vi "Diagnostics.Main.UUDT.Engine.vi"(8 "error in (no error)":errorcluster, 11 "State Variables":T1={"Comm"=refnum, "Parameters"={"Name"="", "CAN"={"Interface"="", "Baud Rate"=0, "Diagnostic Protocol"=enum."GMLAN", "Transport Protocol"=enum."ISO TP - Normal Mode", "Transmit ID"=0, "Receive ID"=2, "Transmit Extension"=1, "Receive Extension"=255, "Receive UUDT ID"=0, "Enable Stream"=TRUE, "VW TP Channel ID"=1, "Fill Frame"=FALSE, "Fill Byte"=0, "Termination"=FALSE, "LIN Cluster"="", "NAD"=8, "IO Mode"=0, "Max DLC"=0, "FD Baud Rate"=2, "Timeout"=1}, "986x"={"Enable"=FALSE, "RIO Device"="", "Bitfile"=path ""}, "Reads"=[], "Frames Lookup"=variant(enum16{"GMLAN", "KWP-2000", "UDS"} enum."GMLAN"), "Writes"=[], "DPIDs"=[], "DPID Lookup"=variant(u32 0), "DTC"={"Descriptor"={"DTC Byte Length"=1, "Status Byte Length"=1, "Add Data Byte Length"=1, "Byte Order"=enum."Motorola"}, "Value.Code"=[], "Value.String"=[], "Value.J2012String"=[], "Status.Code"=[], "Status.String"=[]}, "Created DTCs"=0, "Polls"=[], "Service Channels Status Lookup"=variant, "Trigger Lookup"=variant, "Security"={"Type"=enum."None", "Source DLL Path"=path "", "Target DLL Path"=path "", "Security Level"=0}}, "ADCS Connection"={"Diag CAN Handle"=0, "Transport Protocol"=enum."ISO TP - Normal Mode", "Receive Address Extension"=0, "Transmit Address Extension"=0, "Receive CAN Id"=0, "Transmit CAN Id"=0, "Log Frames ?"=FALSE, "My TP Address"=0, "Other TP Address"=0, "T1"=0, "T2"=0, "T3"=0, "T4"=0, "Tx SN"=0, "Block Size"=0, "Rx SN"=0, "VW TP Initialized?"=FALSE, "Tx block no"=0, "baud rate"=0, "Interface"="", "Channel Diag CAN Handle"=0, "UDP Connection ID"=refnum, "TCP Connection ID"=refnum, "Target IP Addr"=0, "Source Address"=0, "Target Address"=0, "Send Header NACK?"=FALSE, "DLL Handle"=0, "NAD"=0, "Time Stamp read first"=0.0, "Time Stamp read last"=0.0, "Time Stamp write first"=0.0, "Time Stamp write last"=0.0, "Time Stamp write"=0.0, "Time Stamp read"=0.0, " I/O Mode"=0, "FD Baudrate"=0, "TX_DL"=8, "RX_DL"=8, "DoIP Protocol Version"=1, " Selected I/O Mode"=0, "TesterPresent Counter"=0, "TesterPresent Limit"=0, "TesterPresent Tick[ms]"=10, "TesterPresent RequireResponse?"=FALSE, "TesterPresent Stored Ref?"=FALSE, "TesterPresent Message"=[], "TesterPresent Task Handle"=0, "TesterPresent Semaphore"=refnum, "Response Plausibility Check"=1, "Default Version?"=TRUE, "Diagostic Globals"={"Timeout FC (Bs)"=250, "Timeout CF (Cr)"=250, "Timeout Diag Command"=1000, "Receive Block Size (BS)"=0, "Wait Time CF (STmin)"=5, "Max Waits (N_WFTmax)"=10, "Waits to Send (N_WAIT)"=0, "Time between Waits (TW)"=25, "Fill CAN Frames?"=TRUE, "Fill Byte"=255, "Invalid Response as Error?"=FALSE, "Max RspPending Count"=5, "VWTP Command Timeout"=50, "Transport Protocol"=enum."Diagnostics on IP", "Diag CAN Handle"=0, "DLL Handle"=0, "Timeout RspPending"=1000}, "Session-based Properties?"=FALSE}, "XNET References"={"Database"="", "GMLAN DPID Session"="", "Cluster"=""}, "XNETEngine (GMLAN)"=refnum, "Process"=refnum, "Reads"=refnum, "Writes"=refnum, "Cmds"=refnum, "DTCs"=refnum, "DTC Count"=refnum, "Status"=refnum, "Triggers"=refnum, "CANConnected"=refnum, "LocalStop"=refnum, "LocalCommStatus"=refnum, "Service Channels Status"=refnum, "Settings"=refnum} {"ADCS Connection"."Diagostic Globals"."Fill Byte" format="%x"; "ADCS Connection"."TesterPresent Message" format="%.0x"; "ADCS Connection"."Selected I/O Mode" items=["CAN", "CAN FD", "CAN FD+BRS", "ECU Determined"]; "ADCS Connection"."DoIP Protocol Version" items=["2010"=1, "2012"=2]; "ADCS Connection"."RX_DL" items=["8"=8, "12"=12, "16"=16, "20"=20, "24"=24, "32"=32, "48"=48, "64"=64]; "ADCS Connection"."TX_DL" items=["8"=8, "12"=12, "16"=16, "20"=20, "24"=24, "32"=32, "48"=48, "64"=64]; "ADCS Connection"."I/O Mode" items=["CAN", "CAN FD", "CAN FD+BRS", "Not yet determined"]; "Parameters"."Writes"."Signals"."Byte Order" items=["Little Endian", "Big Endian"]; "Parameters"."Writes"."Signals"."Data Type" items=["Signed", "Unsigned", "IEEE Float"]; "Parameters"."CAN"."IO Mode" items=["CAN 2.0", "CAN FD", "CAN FD+BRS"]; "Parameters"."CAN"."Fill Byte" format="%.0x"; "Parameters"."CAN"."VW TP Channel ID" format="%.0x"; "Parameters"."CAN"."Receive UUDT ID" format="%.0x"; "Parameters"."CAN"."Receive Extension" format="%.0x"; "Parameters"."CAN"."Transmit Extension" format="%.0x"; "Parameters"."CAN"."Receive ID" format="%.0x"; "Parameters"."CAN"."Transmit ID" format="%.0x"; "Parameters"."Reads"."Signals"."Byte Order" items=["Little Endian", "Big Endian"]; "Parameters"."Reads"."Signals"."Data Type" items=["Signed", "Unsigned", "IEEE Float"]}) -> (0 "error out":errorcluster)   [LabVIEW 2019, in "Diagnostics Addon Engine.lvlib"]
uses:
  Diagnostics Addon Engine.lvlib
  Types/Diagnostics.State.ctl
  <vilib>/NI/NIVS Inline Async API/_VS Inline Async API/Process/Process.lvclass
  <vilib>/NI/NI VeriStand Addon Network Comm/Engine/VeriStand Comm.lvclass
  Addon Shared/Types/SysDef.Compile.ctl
  Addon Shared/Types/CAN.ctl
  Addon Shared/Types/CAN.Interface.ctl
  Addon Shared/Types/Protocol.ctl
  Addon Shared/Types/Transport.ctl
  Addon Shared/Types/986x.ctl
  Addon Shared/Types/Frame.Compile.ctl
  Addon Shared/Types/Type.ctl
  Addon Shared/Types/Signal.ctl
  Addon Shared/Types/DPID.ctl
  Addon Shared/Types/DPID.Rate.ctl
  Addon Shared/Types/DTC.Settings.ctl
  Addon Shared/Types/DTC.Descriptor.ctl
  Addon Shared/Types/Poll.Compiled.ctl
  Addon Shared/Types/Security.ctl
  Addon Shared/Types/Security.Type.ctl
  <vilib>/Automotive Diagnostic Command Set/Diagnostic Transport.llb/Diag Reference.ctl
  <vilib>/Automotive Diagnostic Command Set/Diagnostic Transport.llb/Transport Protocol Selector.ctl
  <vilib>/Automotive Diagnostic Command Set/Diagnostic Transport.llb/DoIP Protocol Version.ctl
  <vilib>/Automotive Diagnostic Command Set/Diagnostic Transport.llb/Diag Globals.ctl
  Types/XNET.Refs.ctl
  <vilib>/NI/AMC/Message Queue.ctl
  <vilib>/NI/AMC/Message.ctl
  <vilib>/NI/Tools/Keyed Array/KeyedArray.ctl
  <vilib>/NI/NIVS Inline Async API/_Data Access Engine/Data Access Engine/Types/Write.DVR.ctl
  <vilib>/NI/NIVS Inline Async API/_Data Access Engine/Access Type Classes/Write/Write.lvclass
  <vilib>/NI/NIVS Inline Async API/_Data Access Engine/Data Access Engine/Types/Read.DVR.ctl
  <vilib>/NI/NIVS Inline Async API/_Data Access Engine/Access Type Classes/Read/Read.lvclass
  <vilib>/NI/NIVS Inline Async API/_Data Access Engine/Data Access Engine/Types/ReadWrite.DVR.ctl
  <vilib>/NI/NIVS Inline Async API/_Data Access Engine/Access Type Classes/ReadWrite/ReadWrite.lvclass
  Addon Shared/Types/DTC.Info.ctl
  Types/DTC.ChangeCount.Info.ctl
  <vilib>/xnet/xnet.llb/XNET Frame CAN.ctl
  <vilib>/xnet/xnet.llb/XNET Frame Type CAN.ctl
  <vilib>/NI/NIVS Inline Async API/_Data Access Engine/Access Type Classes/Write/Write.lvclass/Write.ctl
  Addon Shared/Types/Frame.Data.ctl
  Addon Shared/Types/DPID.Lookup.Info.ctl
  Addon Shared/Types/DPID.Lookup.Info.PID.ctl
  <vilib>/NI/NI VeriStand Addon Network Comm/Engine/VeriStand Comm.lvclass/VeriStand Comm.ctl
  <vilib>/NI/NIVS Inline Async API/_VS Inline Async API/Process/Process.lvclass/Process.ctl
  <vilib>/NI/NIVS Inline Async API/_Data Access Engine/Data Access Engine/Methods/Write.Data.vi
  <vilib>/NI/NIVS Inline Async API/_Data Access Engine/Data Access Engine/Methods/Write.Data.Commit.vi
  <vilib>/NI/NIVS Inline Async API/_Data Access Engine/Access Type Classes/Write/Write.ProcessData.vi
  <vilib>/NI/NIVS Inline Async API/_Data Access Engine/Data Access Engine/Methods/Write.Data.Buffer.vi
  Addon Shared/SubVIs/LookupID.Create.vi
  <vilib>/NI/NIVS Inline Async API/_Data Access Engine/Access Type Classes/Write/Write.Commit.vi
  Support Libraries/GMLAN/Utilities/Convert Raw Data to DTCs.vi
  <vilib>/NI/AMC/Send Local Message.vi
  <vilib>/NI/AMC/Read Termination Message.vi
  <vilib>/NI/NIVS Inline Async API/_VS Inline Async API/Error Handling Process/SubVIs/Error.ConvertArray.vi
  <vilib>/NI/NIVS Inline Async API/_Data Access Engine/Access Type Classes/Write/Write.Buffer.vi
  <vilib>/NI/AMC/Create Single Message.vi
  <vilib>/NI/AMC/Update Message Routing Info.vi
  <vilib>/NI/AMC/Globals.vi
  Addon Shared/SubVIs/Constants.vi
  <vilib>/Utility/SystemLogging/Write to System Log.vi
  <vilib>/xnet/xnet.llb/XNET Convert.vi
  <vilib>/xnet/xnet.llb/XNET Convert (Frame CAN to Signal).vi
  <vilib>/xnet/xnet.llb/XNET Read (Frame CAN).vi
  <vilib>/Automotive Diagnostic Command Set/Diagnostic Protocols.llb/Convert to Phys.vi
  <vilib>/NI/AMC/Send Message.vi
  Addon Shared/Diagnostics Addon Shared.lvlib
  <vilib>/NI/AMC/AMC.lvlib
  Support Libraries/GMLAN/GMLAN.lvlib
  <vilib>/NI/NIVS Inline Async API/_Data Access Engine/Data Access Engine/Data Access Engine.lvclass
  <vilib>/NI/Tools/Keyed Array/Tools_KeyedArray.lvlib
  <vilib>/addons/Automotive Diagnostic Command Set/NI_Automotive Diagnostic Command Set.lvlib
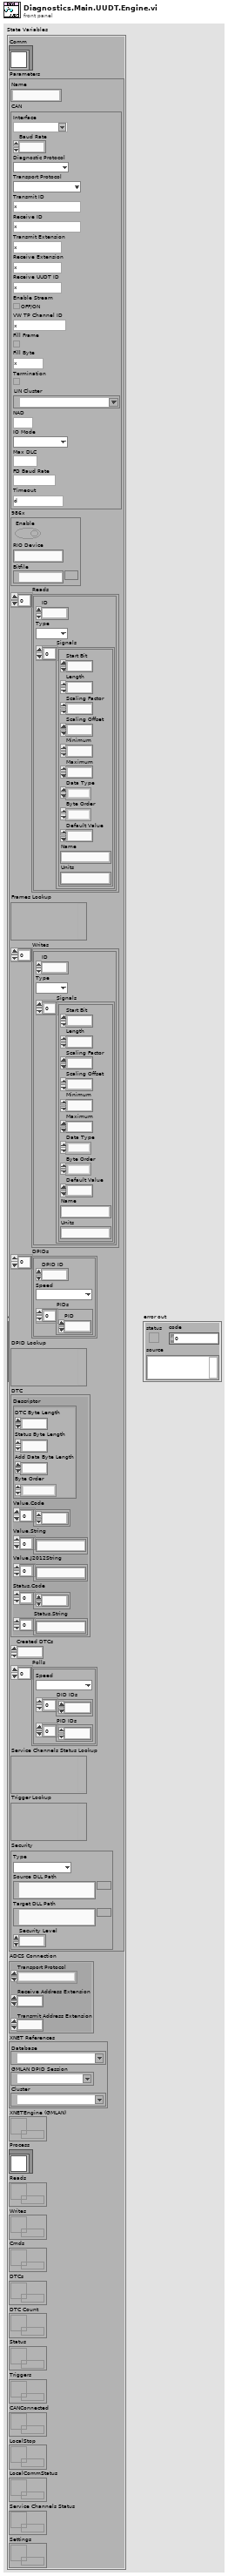
[diagram p1: front panel]
types:
  T1 = typedef "Diagnostics Addon Engine.lvlib/Diagnostics.State.ctl" = cluster{"Comm":refnum<class "VeriStand Comm.lvclass">, "Parameters":T2, "ADCS Connection":T18, "XNET References":T23, "XNETEngine (GMLAN)":T24, "Process":refnum<class "Process.lvclass">, "Reads":T25, "Writes":T26, "Cmds":T27, "DTCs":T25, "DTC Count":T25, "Status":T25, "Triggers":T27, "CANConnected":T25, "LocalStop":refnum<data-value>, "LocalCommStatus":refnum<data-value>, "Service Channels Status":T25, "Settings":T26}
  T2 = typedef "Diagnostics Addon Shared.lvlib/SysDef.Compile.ctl" = cluster{"Name":string, "CAN":T3, "986x":T7, "Reads":T8[], "Frames Lookup":variant, "Writes":T8[], "DPIDs":T11[], "DPID Lookup":variant, "DTC":T13, "Created DTCs":u32, "Polls":T15[], "Service Channels Status Lookup":variant, "Trigger Lookup":variant, "Security":T16}
  T3 = typedef "Diagnostics Addon Shared.lvlib/CAN.ctl" = cluster{"Interface":T4, "Baud Rate":u64, "Diagnostic Protocol":T5, "Transport Protocol":T6, "Transmit ID":u32, "Receive ID":u32, "Transmit Extension":u8, "Receive Extension":u8, "Receive UUDT ID":u32, "Enable Stream":bool, "VW TP Channel ID":u32, "Fill Frame":bool, "Fill Byte":u8, "Termination":bool, "LIN Cluster":refnum<k21>, "NAD":u8, "IO Mode":u32, "Max DLC":u16, "FD Baud Rate":u64, "Timeout":u32}
  T4 = typedef "Diagnostics Addon Shared.lvlib/CAN.Interface.ctl" = string
  T5 = typedef "Diagnostics Addon Shared.lvlib/Protocol.ctl" = enum16{"GMLAN", "KWP-2000", "UDS", "User-Defined"}
  T6 = typedef "Diagnostics Addon Shared.lvlib/Transport.ctl" = enum16{"ISO TP - Normal Mode", "ISO TP - Mixed Mode", "VW TP 2.0", "Diagnostics on IP", "ISO TP LIN"}
  T7 = typedef "Diagnostics Addon Shared.lvlib/986x.ctl" = cluster{"Enable":bool, "RIO Device":string, "Bitfile":path}
  T8 = typedef "Diagnostics Addon Shared.lvlib/Frame.Compile.ctl" = cluster{"ID":u32, "Type":T9, "Signals":T10[]}
  T9 = typedef "Diagnostics Addon Shared.lvlib/Type.ctl" = enum16{"DID", "CDID", "PID", "CPID", "Read Memory", "Write Memory", "IO Control", "Routine Start", "Routine Request", "Routine Stop", "User Defined", "DTC Control", "Clear DTCs", "Read DTCs", "Start DTCs", "DTC Change Count", "Tester Present", "Unlock ECU", "Reset ECU", "Diag Session Control", "Communication Control", "DPID Control", "Poll Control", "Diag CAN Control"}
  T10 = typedef "Diagnostics Addon Shared.lvlib/Signal.ctl" = cluster{"Start Bit":u32, "Length":u32, "Scaling Factor":dbl, "Scaling Offset":dbl, "Minimum":dbl, "Maximum":dbl, "Data Type":u32, "Byte Order":u32, "Default Value":dbl, "Name":string, "Units":string}
  T11 = typedef "Diagnostics Addon Shared.lvlib/DPID.ctl" = cluster{"DPID ID":u8, "Speed":T12, "PIDs":u16[]}
  T12 = typedef "Diagnostics Addon Shared.lvlib/DPID.Rate.ctl" = enum16{"Slow", "Medium", "Fast"}
  T13 = typedef "Diagnostics Addon Shared.lvlib/DTC.Settings.ctl" = cluster{"Descriptor":T14, "Value.Code":dbl[], "Value.String":string[], "Value.J2012String":string[], "Status.Code":dbl[], "Status.String":string[]}
  T14 = typedef "Diagnostics Addon Shared.lvlib/DTC.Descriptor.ctl" = cluster{"DTC Byte Length":i32, "Status Byte Length":i32, "Add Data Byte Length":i32, "Byte Order":enum16{"Motorola", "Intel"}}
  T15 = typedef "Diagnostics Addon Shared.lvlib/Poll.Compiled.ctl" = cluster{"Speed":T12, "DID IDs":u32[], "PID IDs":u32[]}
  T16 = typedef "Diagnostics Addon Shared.lvlib/Security.ctl" = cluster{"Type":T17, "Source DLL Path":path, "Target DLL Path":path, "Security Level":u8}
  T17 = typedef "Diagnostics Addon Shared.lvlib/Security.Type.ctl" = enum16{"None", "DLL", "MasterKey"}
  T18 = typedef "NI_Automotive Diagnostic Command Set.lvlib/Diag Reference.ctl" = cluster{"Diag CAN Handle":u32, "Transport Protocol":T19, "Receive Address Extension":u8, "Transmit Address Extension":u8, "Receive CAN Id":u32, "Transmit CAN Id":u32, "Log Frames ?":bool, "My TP Address":u8, "Other TP Address":u8, "T1":u16, "T2":u16, "T3":u16, "T4":u16, "Tx SN":u8, "Block Size":u8, "Rx SN":u8, "VW TP Initialized?":bool, "Tx block no":u8, "baud rate":u64, "Interface":string, "Channel Diag CAN Handle":u32, "UDP Connection ID":refnum<k16>, "TCP Connection ID":refnum<k5>, "Target IP Addr":u32, "Source Address":u16, "Target Address":u16, "Send Header NACK?":bool, "DLL Handle":u32, "NAD":u8, "Time Stamp read first":dbl, "Time Stamp read last":dbl, "Time Stamp write first":dbl, "Time Stamp write last":dbl, "Time Stamp write":dbl, "Time Stamp read":dbl, " I/O Mode":u32, "FD Baudrate":u64, "TX_DL":u16, "RX_DL":u16, "DoIP Protocol Version":T20, " Selected I/O Mode":u32, "TesterPresent Counter":u32, "TesterPresent Limit":u32, "TesterPresent Tick[ms]":i32, "TesterPresent RequireResponse?":bool, "TesterPresent Stored Ref?":bool, "TesterPresent Message":u8[], "TesterPresent Task Handle":i32, "TesterPresent Semaphore":T21, "Response Plausibility Check":u32, "Default Version?":bool, "Diagostic Globals":T22, "Session-based Properties?":bool}
  T19 = typedef "NI_Automotive Diagnostic Command Set.lvlib/Transport Protocol Selector.ctl" = enum16{"ISO TP - Normal Mode", "ISO TP - Mixed Mode", "VW TP 2.0", "Diagnostics on IP", "ISO TP LIN"}
  T20 = typedef "NI_Automotive Diagnostic Command Set.lvlib/DoIP Protocol Version.ctl" = u8
  T21 = typedef "Semaphore RefNum" = refnum<k1>
  T22 = typedef "NI_Automotive Diagnostic Command Set.lvlib/Diag Globals.ctl" = cluster{"Timeout FC (Bs)":u32, "Timeout CF (Cr)":u32, "Timeout Diag Command":u32, "Receive Block Size (BS)":u8, "Wait Time CF (STmin)":u8, "Max Waits (N_WFTmax)":u8, "Waits to Send (N_WAIT)":i32, "Time between Waits (TW)":u32, "Fill CAN Frames?":bool, "Fill Byte":u32, "Invalid Response as Error?":bool, "Max RspPending Count":u32, "VWTP Command Timeout":u32, "Transport Protocol":T19, "Diag CAN Handle":u32, "DLL Handle":u32, "Timeout RspPending":u32}
  T23 = typedef "Diagnostics Addon Engine.lvlib/XNET.Refs.ctl" = cluster{"Database":refnum<k21>, "GMLAN DPID Session":refnum<k21>, "Cluster":refnum<k21>}
  T24 = typedef "AMC.lvlib/Message Queue.ctl" = refnum<queue>
  T25 = typedef "Data Access Engine.lvlib/Data Access Engine.lvclass/Write.DVR.ctl" = refnum<data-value>
  T26 = typedef "Data Access Engine.lvlib/Data Access Engine.lvclass/Read.DVR.ctl" = refnum<data-value>
  T27 = typedef "Data Access Engine.lvlib/Data Access Engine.lvclass/ReadWrite.DVR.ctl" = refnum<data-value>
  T28 = typedef "Diagnostics Addon Shared.lvlib/DTC.Info.ctl" = cluster{"Timestamp":dbl, "DTC":dbl, "Status":dbl, "Add Data":dbl}
  T29 = typedef "Diagnostics Addon Engine.lvlib/DTC.ChangeCount.Info.ctl" = cluster{"DTCCountChange?":bool, "Timestamp":timestamp}
  T30 = typedef "XNET Frame CAN.ctl" = cluster{"timestamp":timestamp, "payload":u8[], "identifier":u32, "type":T31, "extended?":bool, "echo?":bool}
  T31 = typedef "XNET Frame Type CAN.ctl" = u8
  T32 = cluster{"Change DTC Count Cluster":T29, "Previous DTCs":T28[], "Prev DTC Frames":T30[]}
  T33 = typedef "Diagnostics Addon Shared.lvlib/Frame.Data.ctl" = cluster{"ID":u32, "Raw Frame":u8[], "error out":errorcluster}
  T34 = typedef "Diagnostics Addon Shared.lvlib/DPID.Lookup.Info.ctl" = cluster{"PID Info":T35}
  T35 = typedef "Diagnostics Addon Shared.lvlib/DPID.Lookup.Info.PID.ctl" = cluster{"PID":u16, "Frame Length":u8}
  T36 = typedef "Diagnostic Trouble Code.ctl" = cluster{"DTC":u32, "Status":u32, "Add Data":u32}
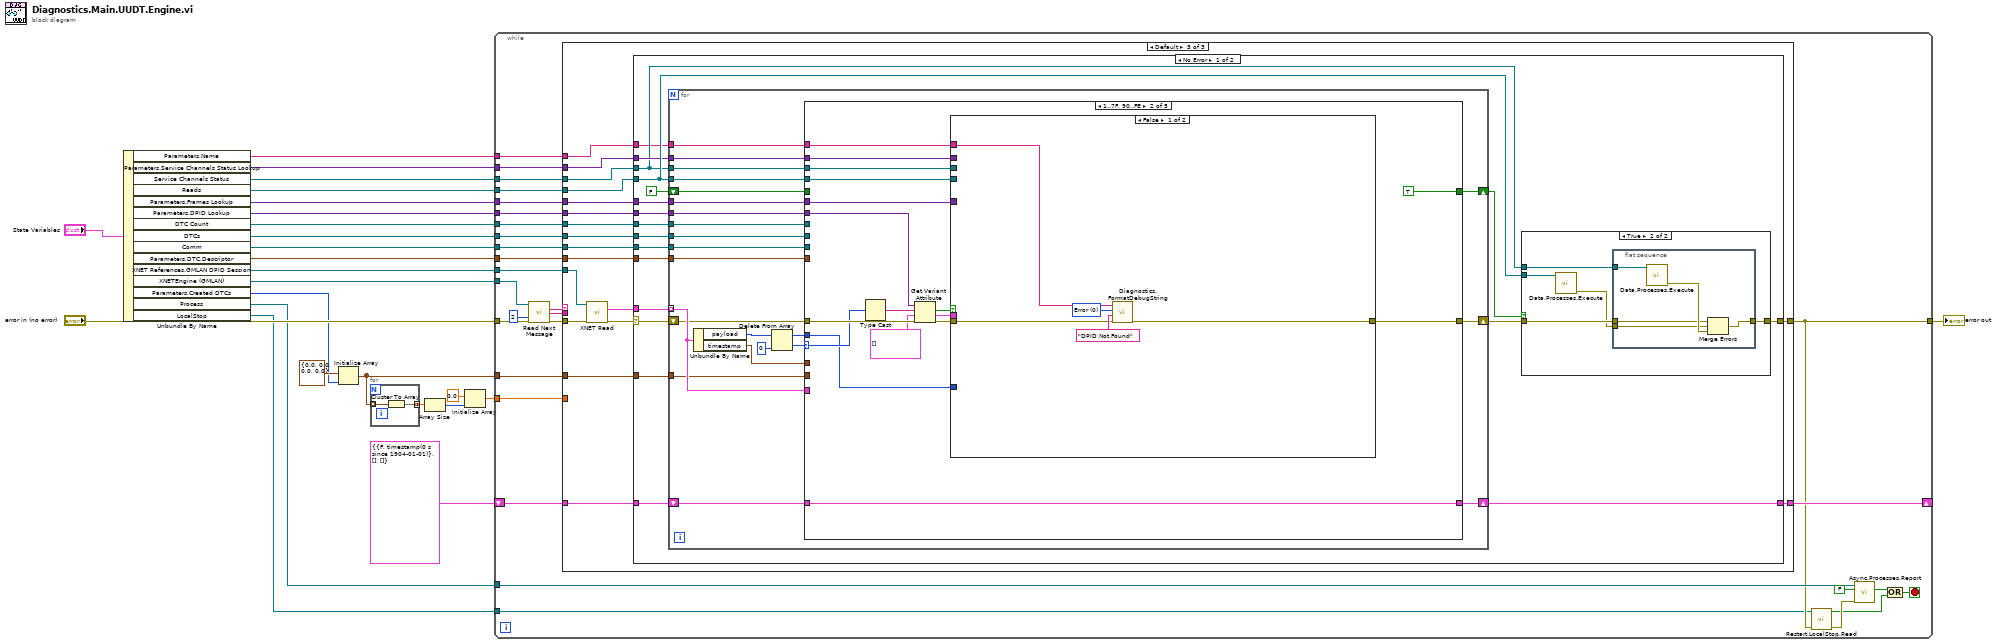
[diagram p0: block diagram]
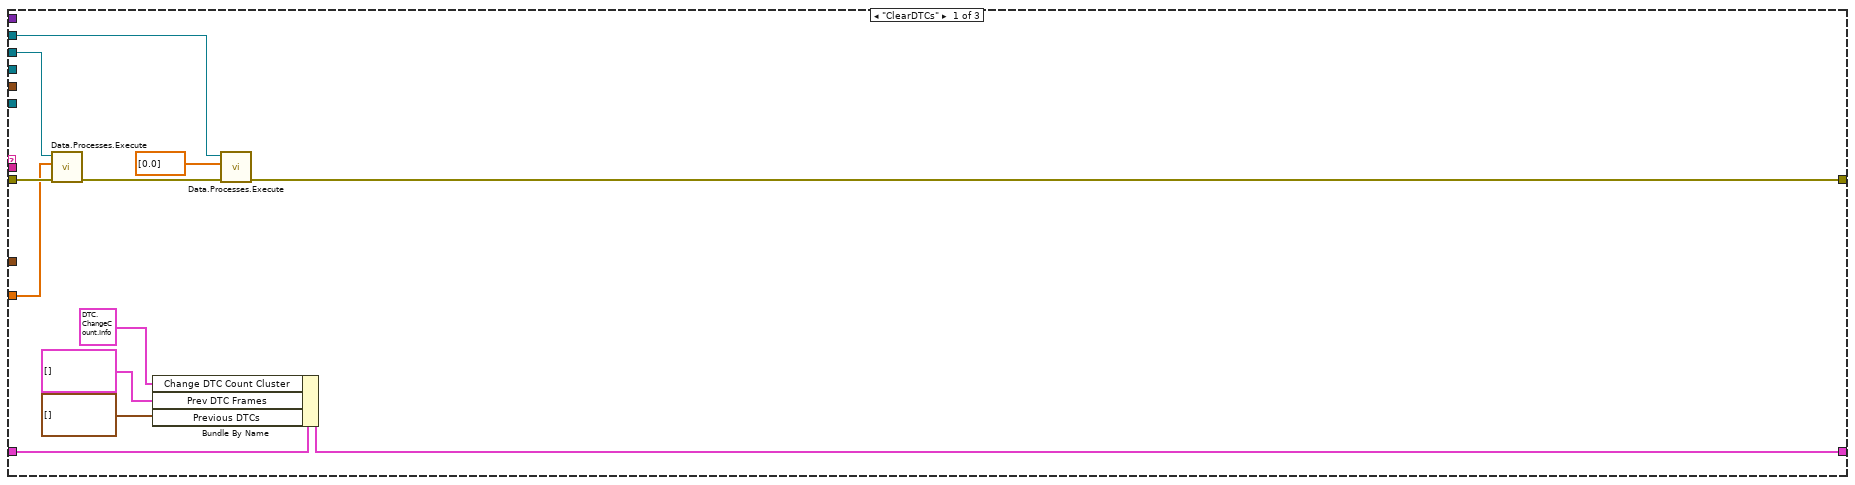
[diagram p2: hidden frame]
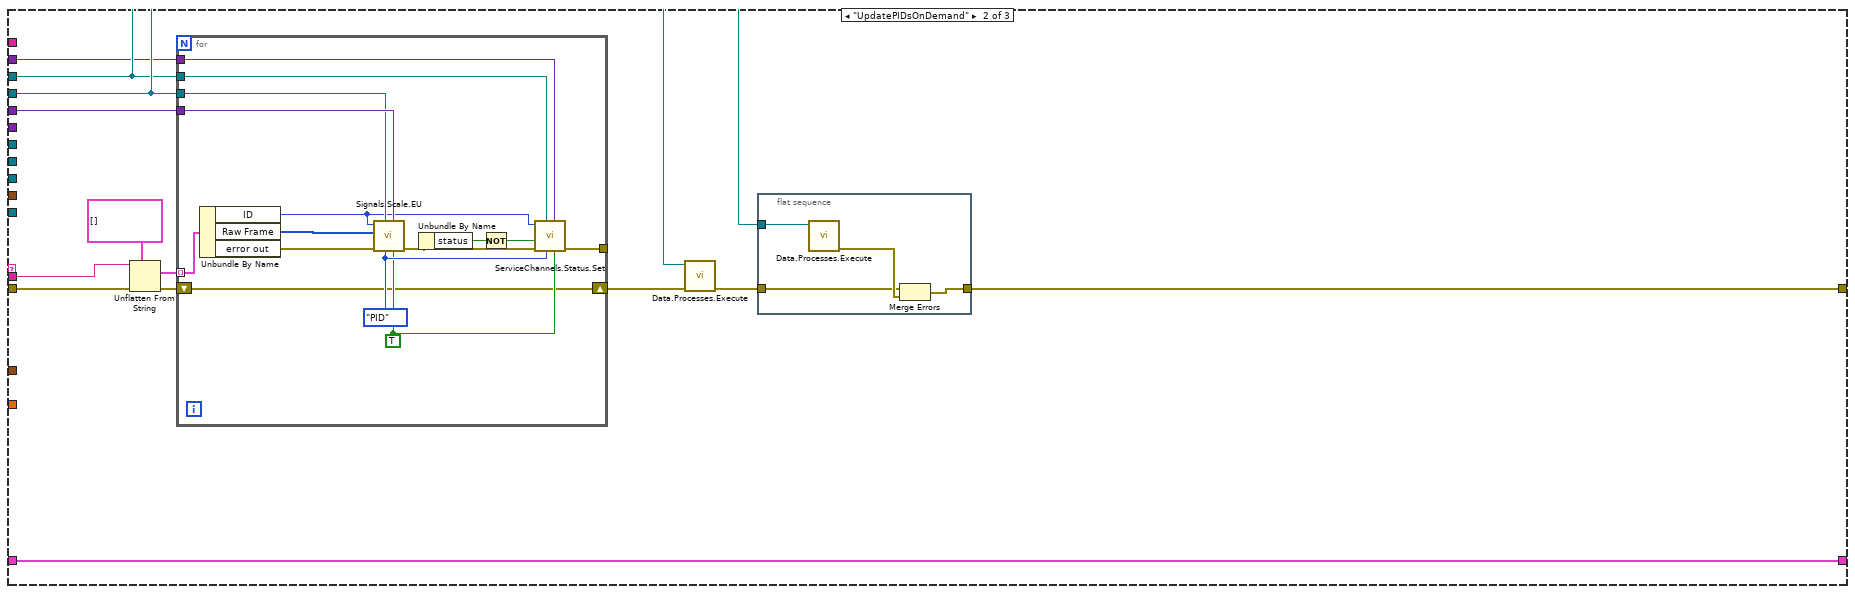
[diagram p3: hidden frame]
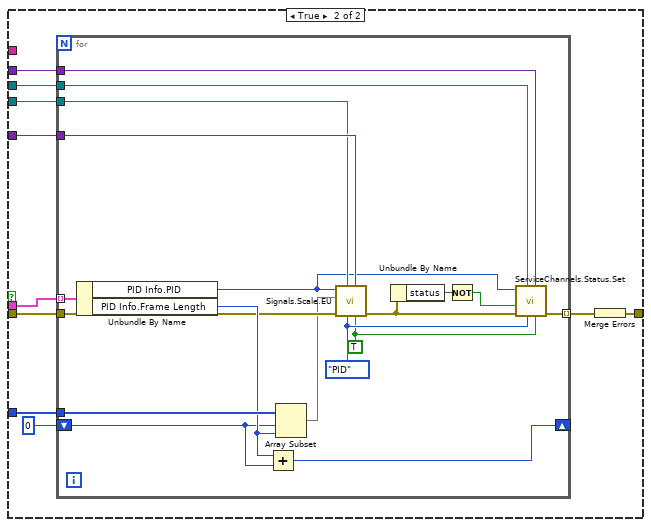
[diagram p5: hidden frame]
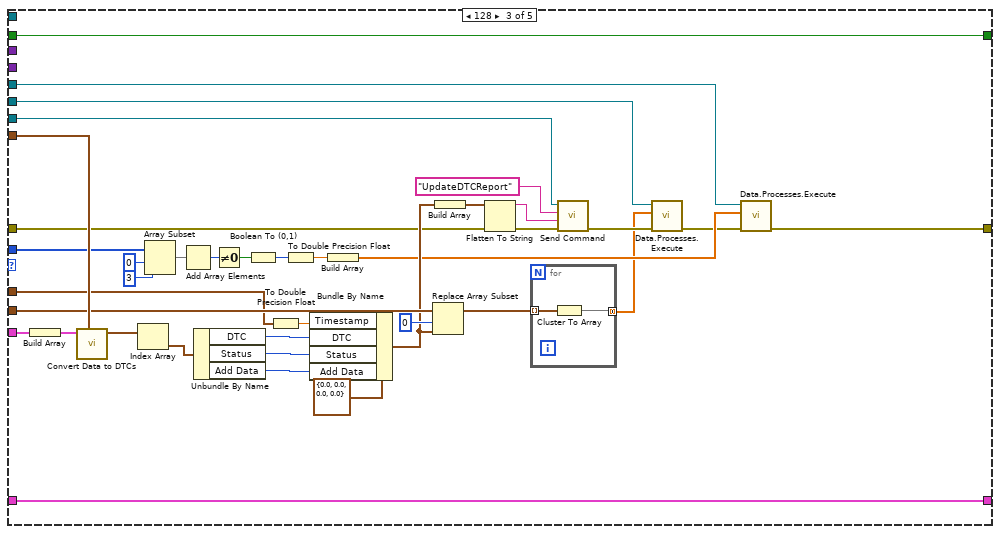
[diagram p6: hidden frame]
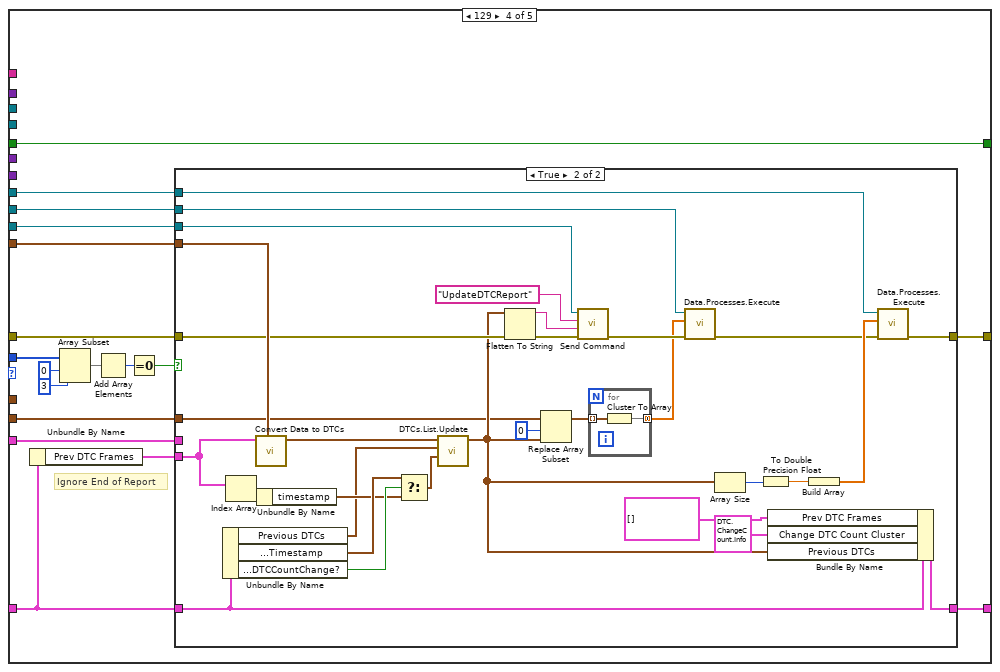
[diagram p7: hidden frame]
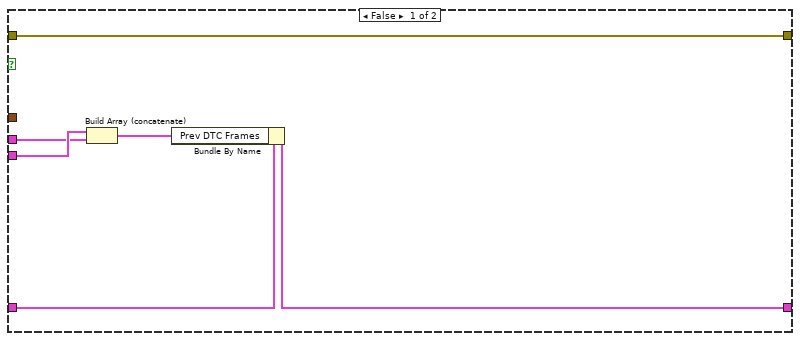
[diagram p8: hidden frame]
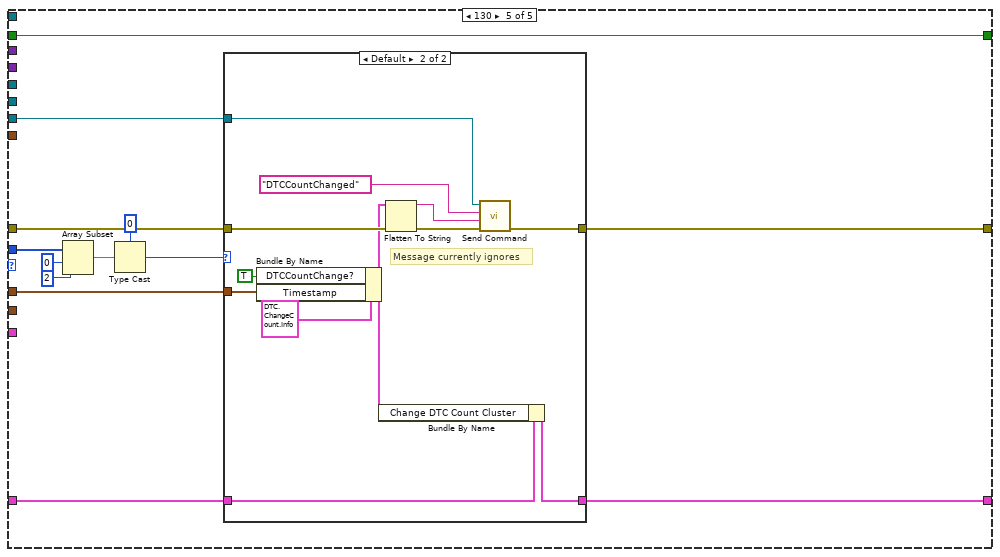
[diagram p9: hidden frame]
diagram:
  n1 = Unbundle By Name("State Variables") -> ("Parameters.Name"=w1:string, "Parameters.Service Channels Status Lookup"=w2:variant, "Service Channels Status"=w3:T25, "Reads"=w20:T25, "Parameters.Frames Lookup"=w19:variant, "Parameters.DPID Lookup"=w13:variant, "DTC Count"=w15:T25, "DTCs"=w23:T25, "Comm"=w22:refnum<class "VeriStand Comm.lvclass">, "Parameters.DTC.Descriptor"=w16:T14, "XNET References.GMLAN DPID Session"=w18:refnum<k21>, "XNETEngine (GMLAN)"=w12:T24, "Parameters.Created DTCs"=w11:u32, "Process"=w5:refnum<class "Process.lvclass">, "LocalStop"=w4:refnum<data-value>)
  n2 = Initialize Array(T28 {"Timestamp"=0.0, "DTC"=0.0, "Status"=0.0, "Add Data"=0.0} ("Diagnostic Trouble Code"), w11) -> (w10:T28[])
  n3 = for {
    tunnel: w10 -> [w27] mode=indexing
    tunnel: [w26] -> w7 mode=concatenating
    n4 = Cluster To Array(cluster=w27) -> (array=w26:dbl[])
  }
  n5 = Array Size(array=w7) -> (size(s)=w8:i32)
  n6 = Initialize Array(0.0 ("element"), w8) -> (w6:dbl[])
  n7 = while {
    tunnel: "error in (no error)" -> [w50]
    tunnel: [w34] -> w17
    tunnel: w16 -> [w56]
    tunnel: w18 -> [w55]
    tunnel: w19 -> [w54]
    tunnel: w20 -> [w53]
    tunnel: w22 -> [w52]
    tunnel: w5 -> [w39]
    tunnel: w12 -> [w44]
    shift-right: [w46] -> _
    shift-left: T32 {"Change DTC Count Cluster"={"DTCCountChange?"=FALSE, "Timestamp"=timestamp(0 s since 1904-01-01)}, "Previous DTCs"=[], "Prev DTC Frames"=[]} -> [w47]
    tunnel: w23 -> [w45]
    tunnel: w15 -> [w43]
    tunnel: w10 -> [w42]
    tunnel: w13 -> [w41]
    tunnel: w6 -> [w36]
    tunnel: w4 -> [w31]
    tunnel: w3 -> [w30]
    tunnel: w2 -> [w29]
    tunnel: w1 -> [w28]
    stop <- w33 stop-if-true
    n8 = call <vilib>:"Read Next Message.vi"("message queue in"=w44, "timeout (1 ms)"=2 ("timeout (1ms)"), "error in"=w50) -> ("message name"=w48:string, "message value"=w40:string, "error out"=w49:errorcluster)  [unwired: 5 in, 5 out]
    n9 = case shown="Default" w48 {
      tunnel: [w59 w69 w116] -> w34
      tunnel: w56 -> [_ _ w115]
      tunnel: w49 -> [w58 w81 w114]
      tunnel: w55 -> [_ _ w113]
      tunnel: w54 -> [_ w76 w112]
      tunnel: w53 -> [_ w73 w111]
      tunnel: w52 -> [_ _ w110]
      tunnel: w47 -> [w68 w75 w109]
      tunnel: [w67 w75 w108] -> w46
      tunnel: w45 -> [w63 _ w107]
      tunnel: w43 -> [w61 _ w106]
      tunnel: w42 -> [_ _ w105]
      tunnel: w41 -> [_ _ w104]
      tunnel: w40 -> [_ w80 _]
      tunnel: w36 -> [w57 _ _]
      tunnel: w30 -> [_ w71 w103]
      tunnel: w29 -> [_ w70 w102]
      tunnel: w28 -> [_ _ w101]
      frame "ClearDTCs" {
        n10 = call-poly <vilib>:"Data.Processes.Execute.vi"("error in (no error)"=w58, "Values"=w57, "Ref"=w63) -> ("error out"=w60:errorcluster)  [unwired: 8 in]
        n11 = Bundle By Name(cluster=w68, "Change DTC Count Cluster"=T29 {"DTCCountChange?"=FALSE, "Timestamp"=timestamp(0 s since 1904-01-01)}, "Prev DTC Frames"=T30[] [] ("Previous DTC Frames"), "Previous DTCs"=T28[] []) -> (w67:T32)
        n12 = call-poly <vilib>:"Data.Processes.Execute.vi"("error in (no error)"=w60, "Values"=dbl[] [0.0] ("element"), "Ref"=w61) -> ("error out"=w59:errorcluster)  [unwired: 8 in]
      }
      frame "UpdatePIDsOnDemand" {
        n13 = Unflatten From String(type=T33[] [], binary string=w80, error in (no error)=w81) -> (value=w77:T33[], error out=w78:errorcluster)  [unwired: 2 in, 1 out]
        n14 = for {
          shift-right: [w96] -> w74
          shift-left: w78 -> [w96]
          tunnel: w77 -> [w100] mode=indexing
          tunnel: w76 -> [w92]
          tunnel: w73 -> [w91]
          tunnel: w71 -> [w93]
          tunnel: w70 -> [w94]
          tunnel: [w95] -> _
          w98 = TRUE ("Buffer?")
          w99 = Type."PID" ("Type")
          n15 = Unbundle By Name(w100) -> ("ID"=w90:u32, "Raw Frame"=w86:u8[], "error out"=w97:errorcluster)
          n16 = call "Signals.Scale.EU.vi"("Buffer?"=w98, "Lookup"=w92, "Type"=w99, "Reads Ref"=w91, "error in (no error)"=w97, "Unscaled Data"=w86, "ID"=w90) -> ("error out"=w89:errorcluster)  [unwired: 4 in]
          n17 = Unbundle By Name(w89) -> ("status"=w88:bool)
          n18 = Not(x=w88) -> (.not. x?=w87:bool)
          n19 = call "ServiceChannels.Status.Set.vi"("Buffer?"=w98, "Status Lookup"=w94, "Type"=w99, "Service Channels Status Ref"=w93, "error in (no error)"=w89, "Status"=w87, "ID"=w90) -> ("error out"=w95:errorcluster)  [unwired: 4 in]
        }
        n20 = call-poly <vilib>:"Data.Processes.Execute.vi"("error in (no error)"=w74, "Ref"=w73) -> ("error out"=w72:errorcluster)  [unwired: 9 in]
        n21 = flat-sequence {
          tunnel: w72 -> [w83]
          tunnel: w71 -> [w85]
          tunnel: [w82] -> w69
          frame #0 {
            n22 = call-poly <vilib>:"Data.Processes.Execute.vi"("Ref"=w85) -> ("error out"=w84:errorcluster)  [unwired: 10 in]
            n23 = Merge Errors(w83, w84) -> (w82:errorcluster)
          }
        }
      }
      frame Default {
        n24 = call-poly <vilib>:"XNET Read.vi"("session in"=w113, "error in (no error)"=w114) -> ("data"=w117:T30[], "error out"=w118:errorcluster)  [unwired: 10 in, 2 out]
        n25 = case shown="No Error" w118 {
          selector: w118 -> [w136 w350]
          tunnel: w117 -> [w137 _]
          tunnel: [w132 w350] -> w116
          tunnel: w115 -> [w134 _]
          tunnel: w112 -> [w133 _]
          tunnel: w111 -> [w122 _]
          tunnel: w110 -> [w131 _]
          tunnel: w109 -> [w128 w349]
          tunnel: [w127 w349] -> w108
          tunnel: w107 -> [w126 _]
          tunnel: w106 -> [w125 _]
          tunnel: w105 -> [w124 _]
          tunnel: w104 -> [w123 _]
          tunnel: w103 -> [w120 _]
          tunnel: w102 -> [w121 _]
          tunnel: w101 -> [w119 _]
          frame No Error {
            n26 = for {
              tunnel: w137 -> [w160] mode=indexing
              shift-right: [w142] -> w135
              shift-left: w136 -> [w143]
              tunnel: w134 -> [w159]
              tunnel: w133 -> [w158]
              tunnel: w131 -> [w157]
              shift-right: [w154] -> w129
              shift-left: FALSE -> [w155]
              shift-right: [w153] -> w127
              shift-left: w128 -> [w152]
              tunnel: w126 -> [w151]
              tunnel: w125 -> [w150]
              tunnel: w124 -> [w149]
              tunnel: w123 -> [w148]
              tunnel: w122 -> [w141]
              tunnel: w120 -> [w140]
              tunnel: w121 -> [w139]
              tunnel: w119 -> [w138]
              n27 = Unbundle By Name(w160) -> ("payload"=w146:u8[], "timestamp"=w156:timestamp)
              n28 = Delete From Array(array=w146, index=0) -> (deleted portion=w144:u8, array with subset deleted=w145:u8[])  [unwired: 1 in]
              n29 = case shown="1..7F, 90..FE" w144 {
                selector: w144 -> [_ w170 _ _ _]
                tunnel: w145 -> [_ w167 w242 w271 w321]
                tunnel: w160 -> [_ _ w251 w255 _]
                tunnel: [w163 w180 w216 w263 w318] -> w142
                tunnel: w143 -> [w163 w177 w221 w264 w317]
                tunnel: w159 -> [_ _ w249 w265 _]
                tunnel: w158 -> [_ w168 _ _ _]
                tunnel: w157 -> [_ _ w224 w258 w311]
                tunnel: w156 -> [_ _ w229 _ w316]
                tunnel: w155 -> [w162 _ w248 w260 w315]
                tunnel: [w162 TRUE w248 w260 w315] -> w154
                tunnel: [w161 w178 w247 w262 w313] -> w153
                tunnel: w152 -> [w161 w178 w247 w261 w314]
                tunnel: w151 -> [_ _ w220 w259 _]
                tunnel: w150 -> [_ _ w218 w257 _]
                tunnel: w149 -> [_ _ w236 w254 _]
                tunnel: w148 -> [_ w171 _ _ _]
                tunnel: w141 -> [_ w169 _ _ _]
                tunnel: w140 -> [_ w166 _ _ _]
                tunnel: w139 -> [_ w165 _ _ _]
                tunnel: w138 -> [_ w164 _ _ _]
                frame Default {
                }
                frame 1..127, 144..254 {
                  n30 = Type Cast(x=w170) -> (*(type *) &x=w174:string)  [unwired: 1 in]
                  n31 = Get Variant Attribute(Variant=w171, name=w174, default value (empty Variant)=T34[] [], error in=w177) -> (found=w172:bool, value=w175:T34[], error out=w176:errorcluster)  [unwired: 1 out]
                  n32 = case shown="False" w172 {
                    tunnel: [w182 w186] -> w180
                    tunnel: w176 -> [w181 w188]
                    tunnel: w175 -> [_ w195]
                    tunnel: w167 -> [_ w194]
                    tunnel: w169 -> [_ w193]
                    tunnel: w168 -> [_ w192]
                    tunnel: w166 -> [_ w190]
                    tunnel: w165 -> [_ w189]
                    tunnel: w164 -> [w185 _]
                    frame False {
                      w183 = 0 items=["Error", "Warning", "Informational"] ("severity (Informational)")
                      n33 = call "Diagnostics.FormatDebugString.vi"("error in (no error)"=w181, "State"="DPID Not Found" ("Debug String"), "severity (Informational)"=w183, "Name"=w185) -> ("error out"=w182:errorcluster)  [unwired: 7 in]
                    }
                    frame True {
                      n34 = for {
                        tunnel: w195 -> [w213] mode=indexing
                        tunnel: w193 -> [w201]
                        tunnel: w192 -> [w202]
                        tunnel: w194 -> [w212]
                        shift-right: [w209] -> _
                        shift-left: 0 -> [w210]
                        tunnel: w190 -> [w203]
                        tunnel: w189 -> [w204]
                        tunnel: w188 -> [w206]
                        tunnel: [w205] -> w187 mode=indexing
                        w207 = TRUE ("Buffer?")
                        w208 = Type."PID" ("Type")
                        n35 = Unbundle By Name(w213) -> ("PID Info.PID"=w200:u16, "PID Info.Frame Length"=w211:u8)
                        n36 = Add(x=w211, y=w210) -> (x+y=w209:i32)
                        n37 = Array Subset(array=w212, index=w210, length=w211) -> (w196:u8[])
                        n38 = call "Signals.Scale.EU.vi"("Buffer?"=w207, "Lookup"=w202, "Type"=w208, "Reads Ref"=w201, "error in (no error)"=w206, "Unscaled Data"=w196, "ID"=w200) -> ("error out"=w199:errorcluster)  [unwired: 4 in]
                        n39 = Unbundle By Name(w199) -> ("status"=w198:bool)
                        n40 = Not(x=w198) -> (.not. x?=w197:bool)
                        n41 = call "ServiceChannels.Status.Set.vi"("Buffer?"=w207, "Status Lookup"=w204, "Type"=w208, "Service Channels Status Ref"=w203, "error in (no error)"=w199, "Status"=w197, "ID"=w200) -> ("error out"=w205:errorcluster)  [unwired: 4 in]
                      }
                      n42 = Merge Errors(w187) -> (w186:errorcluster)
                    }
                  }
                }
                frame 128 {
                  n43 = Build Array(w251) -> (w250:T30[])
                  n44 = call "Convert Data to DTCs.vi"("DTC descriptor"=w249, "All DTCs"=w250) -> ("DTCs"=w235:T36[])  [unwired: 8 in, 1 out]
                  n45 = Index Array(array=w235) -> (element=w233:T36)  [unwired: 1 in]
                  n46 = Array Subset(array=w242, index=0, length=3) -> (w244:u8[])
                  n47 = Add Array Elements(numeric array=w244) -> (sum=w243:u8)
                  n48 = Unbundle By Name(w233) -> ("DTC"=w230:u32, "Status"=w231:u32, "Add Data"=w232:u32)
                  n49 = Not Equal To 0?(x=w243) -> (x != 0?=w241:bool)
                  n50 = Boolean To (0,1)(Boolean=w241) -> (0, 1=w240:i16)
                  n51 = To Double Precision Float(number=w229) -> (double precision float=w228:dbl)
                  n52 = To Double Precision Float(number=w240) -> (double precision float=w239:dbl)
                  n53 = Bundle By Name(cluster=T28 {"Timestamp"=0.0, "DTC"=0.0, "Status"=0.0, "Add Data"=0.0} ("Diagnostic Trouble Code"), "Timestamp"=w228, "DTC"=w230, "Status"=w231, "Add Data"=w232) -> (w223:T28)
                  n54 = Build Array(w239) -> (w219:dbl[])
                  n55 = Replace Array Subset(array=w236, new element=w223, index=0) -> (w237:T28[])
                  n56 = Build Array(w223) -> (w222:T28[])
                  n57 = Flatten To String(anything=w222, error in (no error)=w221) -> (data string=w225:string, error out=w226:errorcluster)  [unwired: 2 in, 1 out]
                  n58 = for {
                    tunnel: w237 -> [w253] mode=indexing
                    tunnel: [w252] -> w214 mode=concatenating
                    n59 = Cluster To Array(cluster=w253) -> (array=w252:dbl[])
                  }
                  n60 = call <vilib>:"Send Command.vi"("error in (no error)"=w226, "message value"=w225, "message name"="UpdateDTCReport" ("Message Name"), "VeriStand Comm in"=w224) -> ("error out"=w215:errorcluster)  [unwired: 6 in, 1 out]
                  n61 = call-poly <vilib>:"Data.Processes.Execute.vi"("error in (no error)"=w215, "Values"=w214, "Ref"=w220) -> ("error out"=w217:errorcluster)  [unwired: 8 in]
                  n62 = call-poly <vilib>:"Data.Processes.Execute.vi"("error in (no error)"=w217, "Values"=w219, "Ref"=w218) -> ("error out"=w216:errorcluster)  [unwired: 8 in]
                }
                frame 129 {
                  # "Ignore End of Report"
                  n63 = Unbundle By Name(w261) -> ("Prev DTC Frames"=w256:T30[])
                  n64 = Array Subset(array=w271, index=0, length=3) -> (w268:u8[])
                  n65 = Add Array Elements(numeric array=w268) -> (sum=w267:u8)
                  n66 = Equal To 0?(x=w267) -> (x = 0?=w266:bool)
                  n67 = case shown="True" w266 {
                    tunnel: w265 -> [_ w308]
                    tunnel: w258 -> [_ w285]
                    tunnel: w264 -> [w277 w301]
                    tunnel: [w277 w280] -> w263
                    tunnel: w261 -> [w276 w300]
                    tunnel: [w275 w298] -> w262
                    tunnel: w259 -> [_ w283]
                    tunnel: w257 -> [_ w281]
                    tunnel: w256 -> [w274 w288]
                    tunnel: w255 -> [w273 _]
                    tunnel: w254 -> [_ w286]
                    frame False {
                      n68 = Build Array (concatenate)(w274, w273) -> (w272:T30[])
                      n69 = Bundle By Name(cluster=w276, "Prev DTC Frames"=w272) -> (w275:T32)
                    }
                    frame True {
                      n70 = Unbundle By Name(w300) -> ("Previous DTCs"=w291:T28[], "Change DTC Count Cluster.Timestamp"=w296:timestamp, "Change DTC Count Cluster.DTCCountChange?"=w307:bool)
                      n71 = Index Array(array=w288) -> (element=w293:T30)  [unwired: 1 in]
                      n72 = call "Convert Data to DTCs.vi"("DTC descriptor"=w308, "All DTCs"=w288) -> ("DTCs"=w303:T36[])  [unwired: 8 in, 1 out]
                      n73 = Unbundle By Name(w293) -> ("timestamp"=w292:timestamp)
                      n74 = Select(t=w296, s=w307, f=w292) -> (s? t:f=w302:timestamp)
                      n75 = call "DTCs.List.Update.vi"("current time"=w302, "Previous Changed DTCs"=w291, "current DTCs"=w303) -> ("Active DTCs"=w287:T28[])  [unwired: 8 in]
                      n76 = Flatten To String(anything=w287, error in (no error)=w301) -> (data string=w304:string, error out=w305:errorcluster)  [unwired: 2 in, 1 out]
                      n77 = Replace Array Subset(array=w286, new element=w287, index=0) -> (w294:T28[])
                      n78 = call <vilib>:"Send Command.vi"("error in (no error)"=w305, "message value"=w304, "message name"="UpdateDTCReport" ("Message Name"), "VeriStand Comm in"=w285) -> ("error out"=w279:errorcluster)  [unwired: 6 in, 1 out]
                      n79 = for {
                        tunnel: w294 -> [w310] mode=indexing
                        tunnel: [w309] -> w278 mode=concatenating
                        n80 = Cluster To Array(cluster=w310) -> (array=w309:dbl[])
                      }
                      n81 = call-poly <vilib>:"Data.Processes.Execute.vi"("error in (no error)"=w279, "Values"=w278, "Ref"=w283) -> ("error out"=w282:errorcluster)  [unwired: 8 in]
                      n82 = Array Size(array=w287) -> (size(s)=w290:i32)
                      n83 = To Double Precision Float(number=w290) -> (double precision float=w289:dbl)
                      n84 = Bundle By Name(cluster=w300, "Prev DTC Frames"=T30[] [] ("data"), "Change DTC Count Cluster"=T29 {"DTCCountChange?"=FALSE, "Timestamp"=timestamp(0 s since 1904-01-01)}, "Previous DTCs"=w287) -> (w298:T32)
                      n85 = Build Array(w289) -> (w284:dbl[])
                      n86 = call-poly <vilib>:"Data.Processes.Execute.vi"("error in (no error)"=w282, "Values"=w284, "Ref"=w281) -> ("error out"=w280:errorcluster)  [unwired: 8 in]
                    }
                  }
                }
                frame 130 {
                  n87 = Array Subset(array=w321, index=0, length=2) -> (w320:u8[])
                  n88 = Type Cast(type=u16 0 ("length"), x=w320) -> (*(type *) &x=w312:u16)
                  n89 = case shown="Default" w312 {
                    tunnel: [w325 w337] -> w318
                    tunnel: w317 -> [w325 w334]
                    tunnel: w316 -> [_ w333]
                    tunnel: w314 -> [w324 w329]
                    tunnel: [w324 w328] -> w313
                    tunnel: w311 -> [_ w326]
                    frame 0 {
                      # "ChangeDTCCount Disabled."
                    }
                    frame Default {
                      # "Message currently ignores"
                      n90 = Bundle By Name(cluster=T29 {"DTCCountChange?"=FALSE, "Timestamp"=timestamp(0 s since 1904-01-01)} ("Cluster"), "DTCCountChange?"=TRUE, "Timestamp"=w333) -> (w330:T29)
                      n91 = Bundle By Name(cluster=w329, "Change DTC Count Cluster"=w330) -> (w328:T32)
                      n92 = Flatten To String(anything=w330, error in (no error)=w334) -> (data string=w336:string, error out=w335:errorcluster)  [unwired: 2 in, 1 out]
                      n93 = call <vilib>:"Send Command.vi"("error in (no error)"=w335, "message value"=w336, "message name"="DTCCountChanged" ("Message Name"), "VeriStand Comm in"=w326) -> ("error out"=w337:errorcluster)  [unwired: 6 in, 1 out]
                    }
                  }
                }
              }
            }
            n94 = case shown="True" w129 {
              tunnel: w135 -> [w338 w340]
              tunnel: [w338 w342] -> w132
              tunnel: w122 -> [_ w343]
              tunnel: w120 -> [_ w341]
              frame False {
              }
              frame True {
                n95 = call-poly <vilib>:"Data.Processes.Execute.vi"("Ref"=w343) -> ("error out"=w339:errorcluster)  [unwired: 10 in]
                n96 = flat-sequence {
                  tunnel: w340 -> [w346]
                  tunnel: w341 -> [w348]
                  tunnel: [w345] -> w342
                  tunnel: w339 -> [w344]
                  frame #0 {
                    n97 = call-poly <vilib>:"Data.Processes.Execute.vi"("Ref"=w348) -> ("error out"=w347:errorcluster)  [unwired: 10 in]
                    n98 = Merge Errors(w346, w344, w347) -> (w345:errorcluster)
                  }
                }
              }
            }
          }
          frame Error {
          }
        }
      }
    }
    n99 = call "Restart.LocalStop.Read.vi"("error in (no error)"=w34, "Data Value Reference in"=w31) -> ("error out"=w35:errorcluster, "LocalStop"=w32:bool)  [unwired: 8 in]
    n100 = call <vilib>:"Async.Processes.Report.vi"("Error"=w35, "Stop Async on Error?"=FALSE ("Stop on Error?"), "Process in"=w39) -> ("Stop"=w37:bool)  [unwired: 7 in, 1 out]
    n101 = Compound Arithmetic op=OR(w37, w32) -> (w33:bool)
  }
  "error out" <- w17
